vi "getTargetPos.vi"(8 "error in (no error)":errorcluster, 11 "Opt_Selector in":refnum<class "Opt_Selector.lvclass">) -> (0 "error out":errorcluster, 2 "Target Pos":u16, 3 "Opt_Selector out":refnum<class "Opt_Selector.lvclass">)   [LabVIEW 2018, in "Opt_Selector.lvclass"]
uses:
  Opt_Selector.lvclass
  Opt_Selector.lvclass/Opt_Selector.ctl
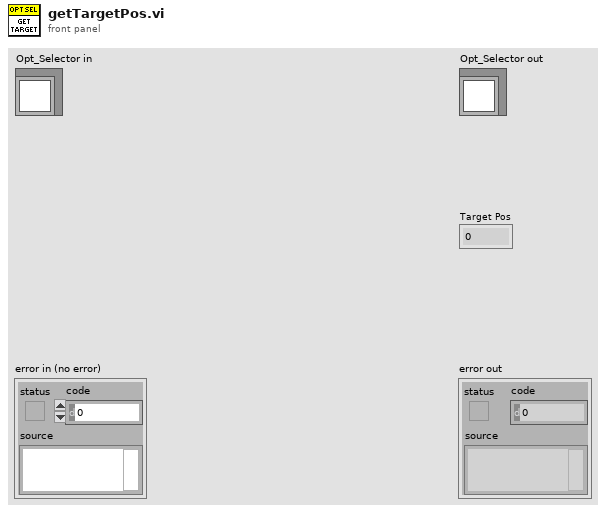
[diagram p1: front panel]
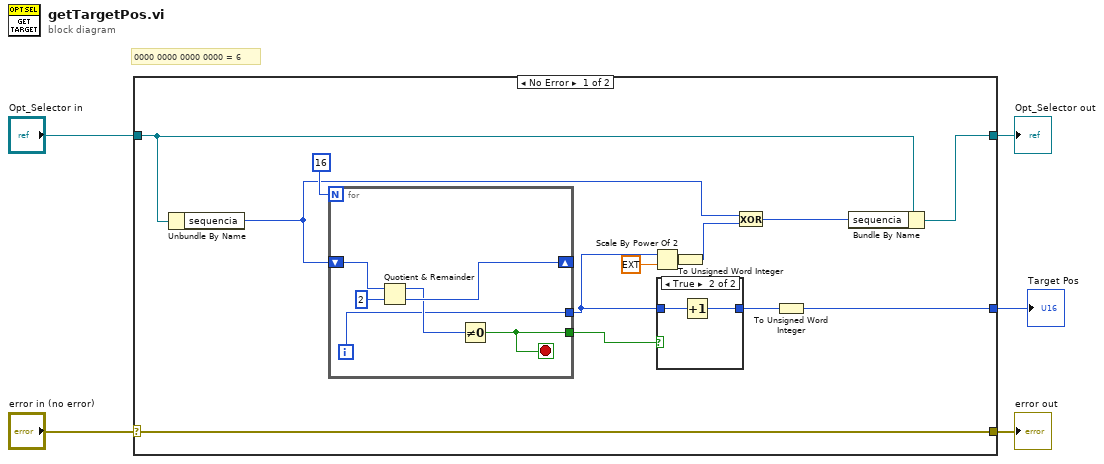
[diagram p0: block diagram]
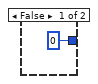
[diagram p2: hidden frame]
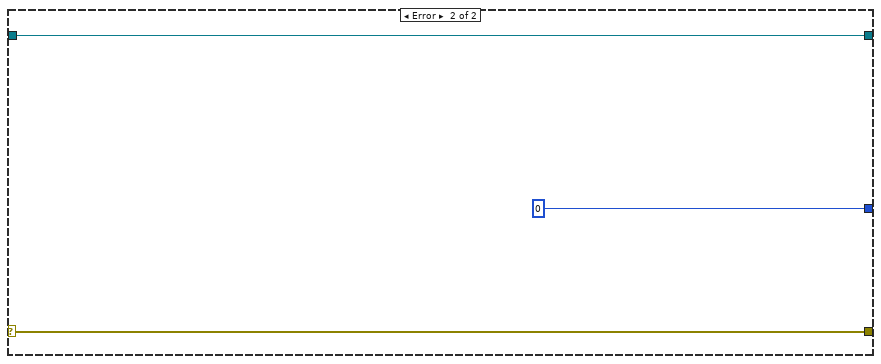
[diagram p3: hidden frame]
diagram:
  # "0000 0000 0000 0000 = 6"
  n1 = case shown="No Error" "error in (no error)" {
    selector: "error in (no error)" -> [w18 w30]
    tunnel: [w18 w30] -> w4
    tunnel: [w17 w29] -> w2
    tunnel: "Opt_Selector in" -> [w10 w29]
    tunnel: [w7 u16 0] -> w1
    frame No Error {
      n2 = Unbundle By Name(w10) -> ("sequencia"=w9:u16)
      n3 = for {
        N: 16 -> [_]
        shift-right: [w25] -> _
        shift-left: w9 -> [w27]
        tunnel: [w23] -> w16
        tunnel: [w22] -> w6
        i -> [w23]
        stop <- w22 stop-if-true
        n4 = Quotient & Remainder(x=w27, y=u16 2) -> (x-y*floor(x/y)=w24:u16, floor(x/y)=w25:u16)
        n5 = Not Equal To 0?(x=w24) -> (x != 0?=w22:bool)
      }
      n6 = Scale By Power Of 2(n=w16, x=ext 1.0) -> (x*2^n=w14:ext)
      n7 = case shown="True" w6 {
        tunnel: w16 -> [_ w21]
        tunnel: [0 w20] -> w8
        frame False {
        }
        frame True {
          n8 = Increment(x=w21) -> (x+1=w20:i32)
        }
      }
      n9 = To Unsigned Word Integer(number=w14) -> (unsigned 16bit integer=w13:u16)
      n10 = Exclusive Or(1:w13, 2:w9) -> (0:w11:u16)
      n11 = To Unsigned Word Integer(number=w8) -> (unsigned 16bit integer=w7:u16)
      n12 = Bundle By Name(cluster=w10, "sequencia"=w11) -> (w17:refnum<class "Opt_Selector.lvclass">)
    }
    frame Error {
    }
  }
  "error out" <- w4
  "Opt_Selector out" <- w2
  "Target Pos" <- w1
